vi "check unsalvageable connection.vi"(8 "error in (no error)":errorcluster, 11 "connection reference":refnum<data-value>) -> (0 "error out":errorcluster)   [LabVIEW 2012, in "TCP Slave.lvclass"]
uses:
  TCP Slave.lvclass
  Connection.ctl
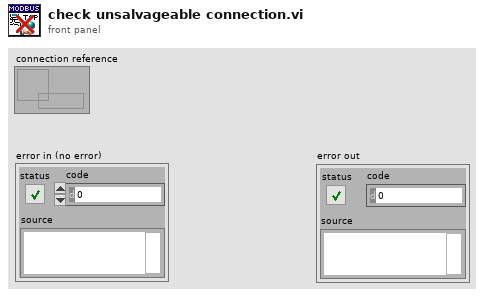
[diagram p1: front panel]
types:
  T1 = typedef "TCP Slave.lvclass/Connection.ctl" = cluster{"Connected?":bool, "IP address":string, "connection error":errorcluster}
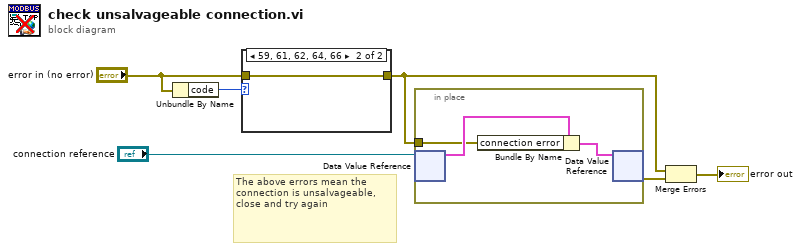
[diagram p0: block diagram]
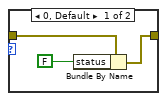
[diagram p2: hidden frame]
diagram:
  # "The above errors mean the connection is unsalvageable, close and try again"
  n1 = Unbundle By Name("error in (no error)") -> ("code"=w6:i32)
  n2 = case shown="59, 61, 62, 64, 66" w6 {
    tunnel: "error in (no error)" -> [w9 w10]
    tunnel: [w7 w10] -> w1
    frame 0, Default {
      n3 = Bundle By Name(cluster=w9, "status"=FALSE) -> (w7:errorcluster)
    }
    frame 59, 61, 62, 64, 66 {
    }
  }
  n4 = in-place {
    in-place-border: w1 -> [w11]
    n5 = in-place-dvr #1("connection reference") -> (w13:T1)  [unwired: 1 out]
    n6 = Bundle By Name(cluster=w13, "connection error"=w11) -> (w12:T1)
    n7 = in-place-dvr #1(w12) -> (w3:errorcluster)  [unwired: 1 out]
  }
  n8 = Merge Errors(w1, w3) -> (→"error out":errorcluster)
